vi "Terminal-PressureSystem-HeaterAlarm-Getter.vi"(8 "error in (no error)":errorcluster caption="错误输入（无错误）", 11 "read operation timeout (ms)":i32=5000 caption="读操作超时（5000毫秒）") -> (0 "error out":errorcluster caption="错误输出", 2 "时间标识":timestamp, 3 "加热装置异常信息":T1)   [LabVIEW 2014]
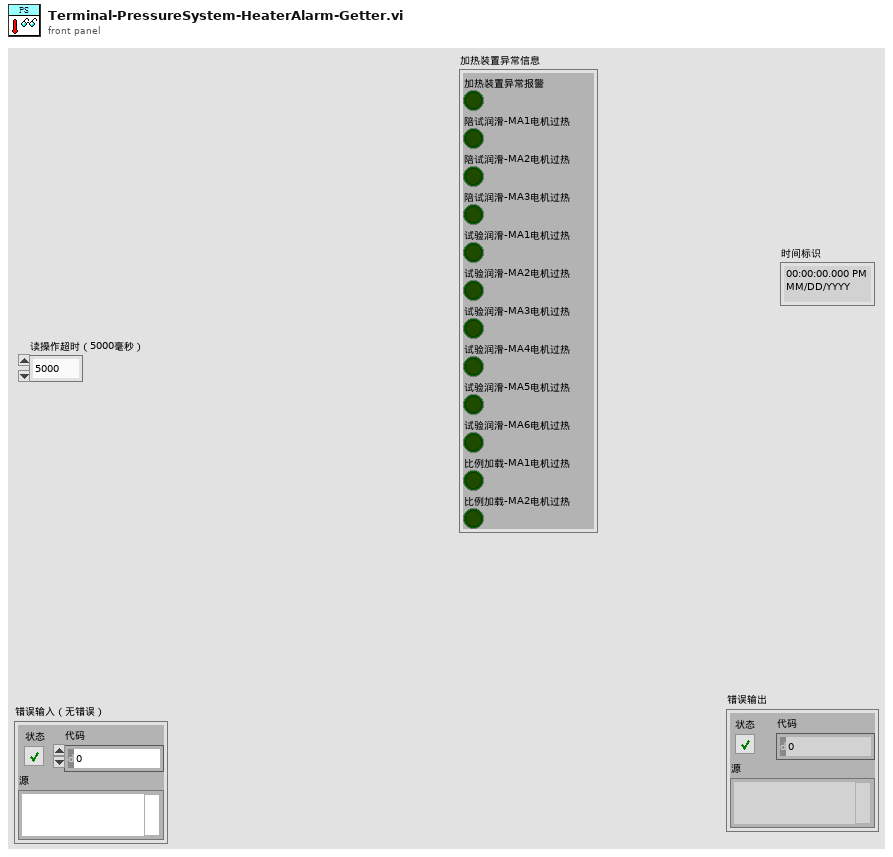
[diagram p1: front panel]
types:
  T1 = cluster{"加热装置异常报警":bool, "陪试润滑-MA1电机过热":bool, "陪试润滑-MA2电机过热":bool, "陪试润滑-MA3电机过热":bool, "试验润滑-MA1电机过热":bool, "试验润滑-MA2电机过热":bool, "试验润滑-MA3电机过热":bool, "试验润滑-MA4电机过热":bool, "试验润滑-MA5电机过热":bool, "试验润滑-MA6电机过热":bool, "比例加载-MA1电机过热":bool, "比例加载-MA2电机过热":bool}
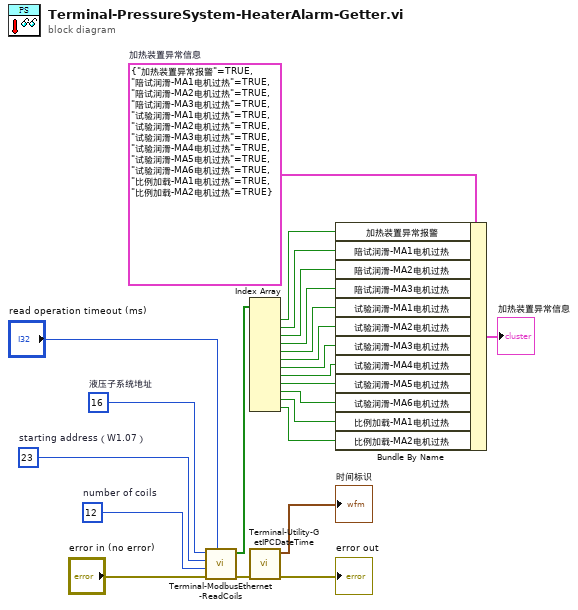
[diagram p0: block diagram]
diagram:
  w11 = T1 {"加热装置异常报警"=TRUE, "陪试润滑-MA1电机过热"=TRUE, "陪试润滑-MA2电机过热"=TRUE, "陪试润滑-MA3电机过热"=TRUE, "试验润滑-MA1电机过热"=TRUE, "试验润滑-MA2电机过热"=TRUE, "试验润滑-MA3电机过热"=TRUE, "试验润滑-MA4电机过热"=TRUE, "试验润滑-MA5电机过热"=TRUE, "试验润滑-MA6电机过热"=TRUE, "比例加载-MA1电机过热"=TRUE, "比例加载-MA2电机过热"=TRUE}  # 加热装置异常信息
  w19 = u16 12  # number of coils
  w20 = u16 23  # starting address（W1.07）
  w9 = u8 16  # 液压子系统地址
  n1 = call "Terminal-ModbusEthernet-ReadCoils.vi"("read operation timeout (ms)"="read operation timeout (ms)", "error in"="error in (no error)", "number of coils"=w19, "starting address"=w20, "unit ID"=w9) -> ("error out"=w21:errorcluster, "coil values"=w18:bool[])  [unwired: 5 in]
  n2 = Index Array(array=w18) -> (element #1=w17:bool, element #2=w16:bool, element #3=w15:bool, element #4=w14:bool, element #5=w13:bool, element #6=w12:bool, element #7=w7:bool, element #8=w6:bool, element #9=w5:bool, element #10=w4:bool, element #11=w3:bool, element #12=w2:bool)  [unwired: 12 in]
  n3 = call "Terminal-Utility-GetIPCDateTime.vi"("error in (no error)"=w21) -> ("error out"=→"error out":errorcluster, "时间标识"=→"时间标识":timestamp)  [unwired: 9 in]
  n4 = Bundle By Name(cluster=w11, "加热装置异常报警"=w17, "陪试润滑-MA1电机过热"=w16, "陪试润滑-MA2电机过热"=w15, "陪试润滑-MA3电机过热"=w14, "试验润滑-MA1电机过热"=w13, "试验润滑-MA2电机过热"=w12, "试验润滑-MA3电机过热"=w7, "试验润滑-MA4电机过热"=w6, "试验润滑-MA5电机过热"=w5, "试验润滑-MA6电机过热"=w4, "比例加载-MA1电机过热"=w3, "比例加载-MA2电机过热"=w2) -> (→"加热装置异常信息":T1)
